vi "NewWindow.vi"   [LabVIEW 2016]
uses:
  <vilib>/regexp/Match Regular Expression.xnode
  Course Project/support/Message Queue/Message Queue.lvlib
panel:
  # "Use Palette \"System\" & Modern\nCreate/Add a copy of this VI in the project"
types:
  T1 = typedef "Message Queue.lvlib/All Message Queues.ctl" = cluster{"IU":refnum<queue>}
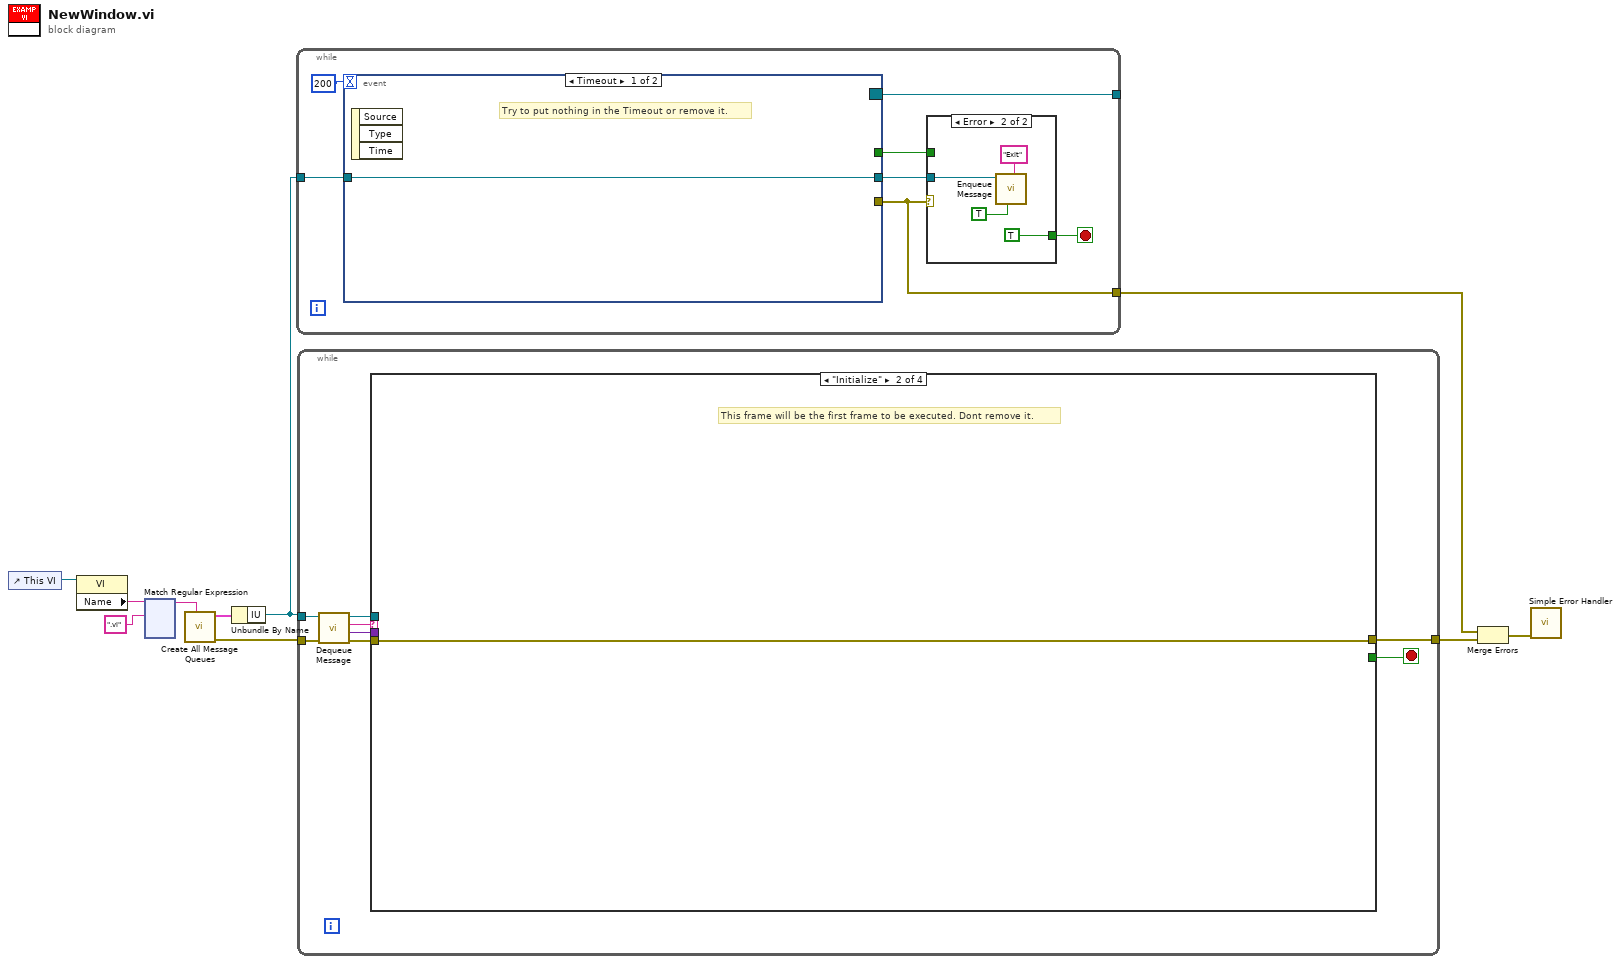
[diagram p0: block diagram]
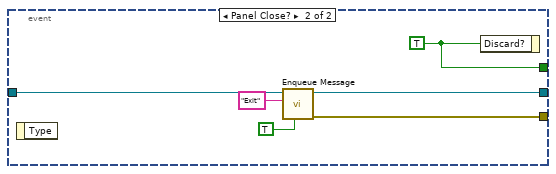
[diagram p3: hidden frame]
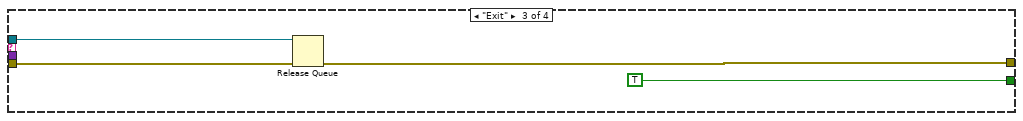
[diagram p5: hidden frame]
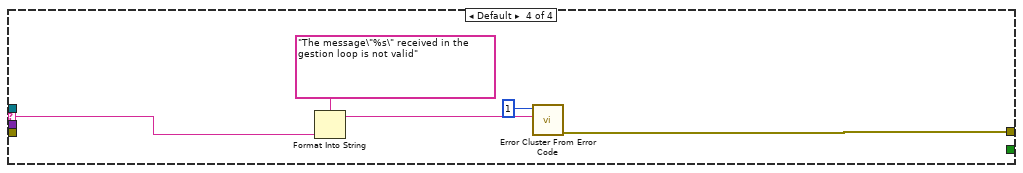
[diagram p6: hidden frame]
diagram:
  n1 = control-ref of="This VI"() -> (w4:refnum<vi>)
  n2 = property class="VI"(reference=w4) -> ("Name"=w3:string)  [unwired: 1 in, 2 out]
  n3 = xnode "Match Regular Expression"("input string"=w3, "regular expression"=".vi") -> ("before match"=w1:string)  [unwired: 4 in, 4 out]
  n4 = call "Create All Message Queues.vi"("QueueName"=w1) -> ("ErrorOut"=w8:errorcluster, "MessageQueueOut"=w10:T1)  [unwired: 9 in]
  n5 = Unbundle By Name(w10) -> ("IU"=w9:refnum<queue>)
  n6 = while {
    tunnel: w9 -> [w17]
    tunnel: [w13] -> w5
    tunnel: [w12] -> _
    stop <- w15 stop-if-true
    n7 = event shown="[0] Timeout" {
      selector: _ -> [_ _]
      dyn-events: [_ _] -> w12
      timeout: 200 -> [_ _]
      tunnel: [_ w29] -> w16
      tunnel: w17 -> [w23 w28]
      tunnel: [_ w27] -> w13
      tunnel: [w23 w26] -> w14
      event Timeout {
        # "Try to put nothing in the Timeout or remove it."
        n8 = event-data() -> ()  [unwired: 1 in, 3 out]
      }
      event Panel Close? {
        w29 = TRUE ("Rejeter ?")
        n9 = event-data() -> ()  [unwired: 1 in, 1 out]
        n10 = call "Enqueue Message.vi"("Prioritary message"=TRUE ("Message prioritaire ? (F)"), "Message"="Exit", "Queue"=w28) -> ("error out"=w27:errorcluster, "Queue dup."=w26:refnum<queue>)  [unwired: 7 in]
        n11 = event-data ("Event Filter Node")("Discard?"=w29) -> ()  [unwired: 1 in, 1 out]
      }
    }
    n12 = case shown="Error" w13 {
      tunnel: [w18 TRUE ("Rejeter ?")] -> w15
      tunnel: w16 -> [w18 _]
      tunnel: w14 -> [_ w21]
      frame No Error {
      }
      frame Error {
        n13 = call "Enqueue Message.vi"("Prioritary message"=TRUE ("Message prioritaire ? (F)"), "Message"="Exit", "Queue"=w21) -> ()  [unwired: 7 in, 2 out]
      }
    }
  }
  n14 = while {
    tunnel: w9 -> [w31]
    tunnel: w8 -> [w35]
    tunnel: [w36] -> w6
    stop <- w37 stop-if-true
    n15 = call "Dequeue Message.vi"("entrée d'erreur (pas d'erreur)"=w35, "File d'attente de messages"=w31) -> ("sortie d'erreur"=w34:errorcluster, "Données de message"=w33:variant, "Message"=w30:string, "File d'attente de message dup."=w32:refnum<queue>)  [unwired: 6 in]
    n16 = case "Conditions des messages" shown="\"Initialize\"" w30 {
      selector: w30 -> [_ _ _ w47]
      tunnel: w32 -> [_ _ w43 _]
      tunnel: w34 -> [w38 w39 w41 _]
      tunnel: [w38 w39 w40 w45] -> w36
      tunnel: [_ _ TRUE _] -> w37
      tunnel: w33 -> [_ _ _ _]
      frame "--------- Initialization ---------" {
      }
      frame "Initialize" {
        # "This frame will be the first frame to be executed. Dont remove it."
      }
      frame "Exit" {
        n17 = Release Queue(queue=w43, error in (no error)=w41) -> (error out=w40:errorcluster)  [unwired: 1 in, 2 out]
      }
      frame Default {
        n18 = Format Into String(format string="The message\"%s\" received in the gestion loop is not valid" ("Texte de message d'erreur inconnu"), w47) -> (resulting string=w44:string)  [unwired: 2 in, 1 out]
        n19 = call <vilib>:"Error Cluster From Error Code.vi"("error message (\"\")"=w44, "error code (0)"=1 ("code d'erreur (0)")) -> ("error out"=w45:errorcluster)  [unwired: 7 in]
      }
    }
  }
  n20 = Merge Errors(w5, w6) -> (w7:errorcluster)
  n21 = call <vilib>:"Simple Error Handler.vi"("error in (no error)"=w7) -> ()  [unwired: 4 in, 5 out]
